vi "Set_Speed.vi"(5 "Channel Name (Calib Tweak)":string, 6 "Calib Tweak":dbl format="%.2f", 7 "Client Name":string, 8 "Channel Name (Volts/Amps)":string, 9 "Demanded Velocity":dbl format="%.2f", 10 "Channel Name (Velocity)":string) -> ()   [LabVIEW 2012]
uses:
  ADAM Client/Sub VIs/ADAM Controls/Update_scan_value.ctl
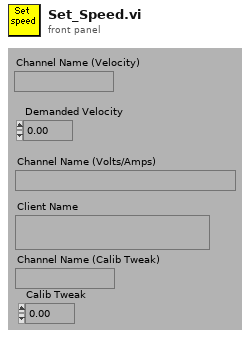
[diagram p1: front panel]
types:
  T1 = enum16{"Append to Global", "Read Global then Clear"}
  T2 = typedef "Update_scan_value.ctl" = cluster{"Channel Name":string, "New Value":dbl}
  T3 = typedef "Ch_description_ADAM.ctl" = cluster{"Ch Name":string, "Type":T4, "Function":T5, "Ch State":T6, "Calibration type":T7, "A":dbl, "B":dbl, "C":dbl, "D":dbl, "Comments":string, "Address":T8, "String":string, "Duty":u16}
  T4 = typedef "Module_type_ADAM.ctl" = string
  T5 = typedef "Function_ADAM.ctl" = enum16{"Analogue Input", "Digital Input", "Event counter", "Event rate", "Analogue Output", "Digital Output", "Relay Output"}
  T6 = typedef "Channel_State.ctl" = enum16{"On", "Off", "Always On", "Always Off"}
  T7 = typedef "Calib_type_ADAM.ctl" = enum16{"Raw", "Bx + A", "Cx^2 + Bx + A", "Dx^3 + Cx^2 + Bx + A", "In Band", "Hi-Tec Q", "Hi-Tec M_dot", "Text"}
  T8 = typedef "Address.ctl" = cluster{"Main":i32, "Ch.":i32, "Sub":i32, "Port Name":string}
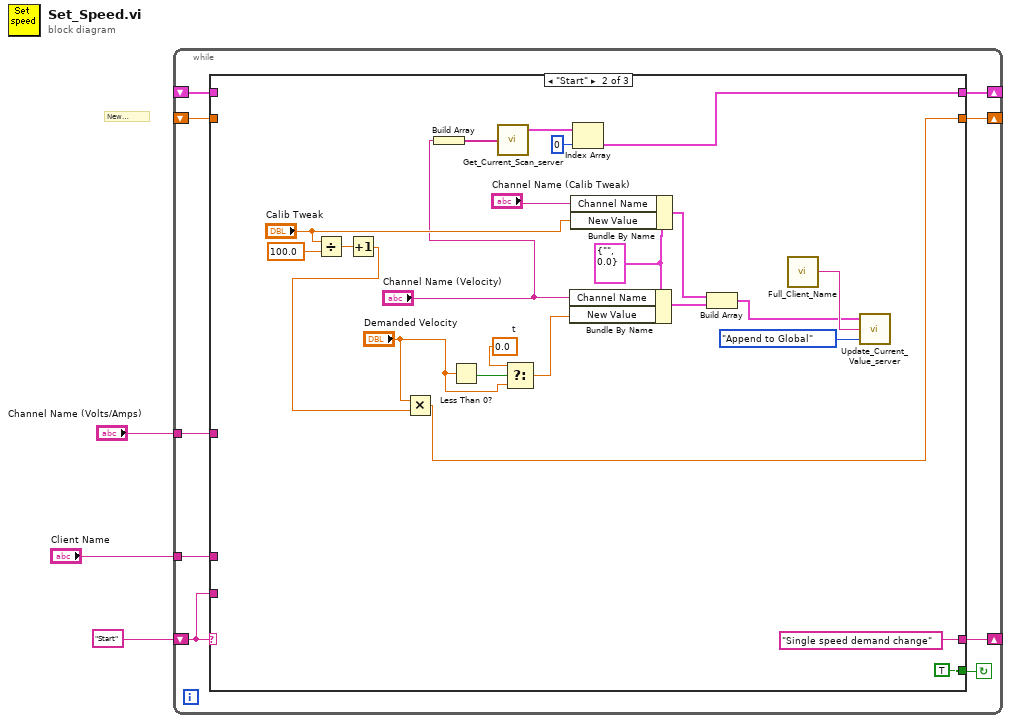
[diagram p0: block diagram]
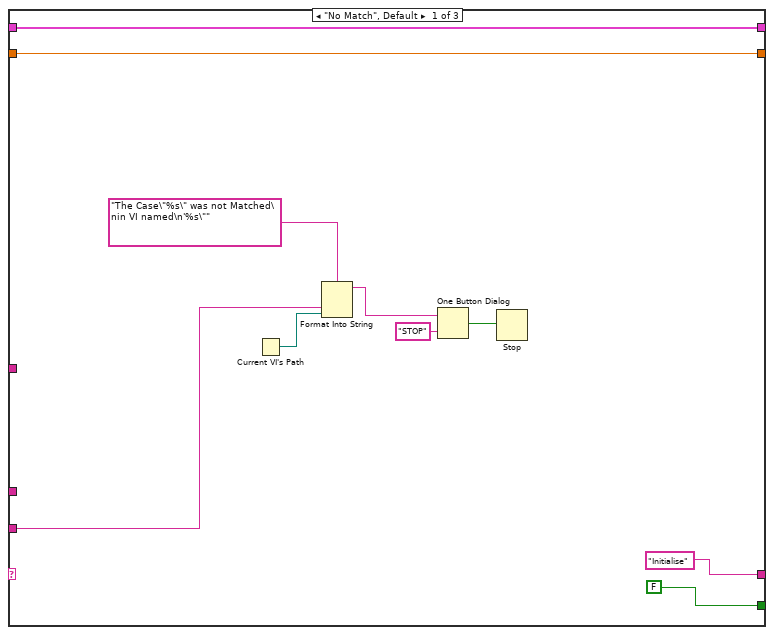
[diagram p2: hidden frame]
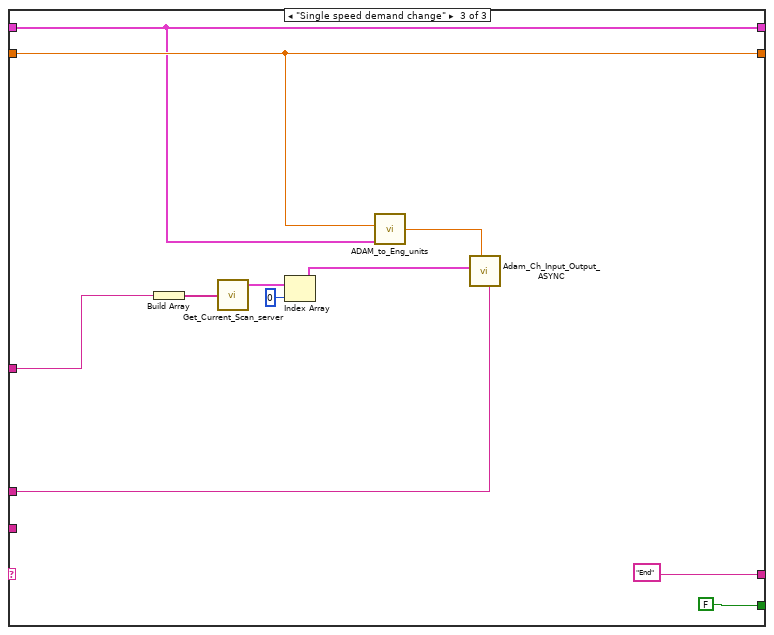
[diagram p3: hidden frame]
diagram:
  # "New Demand"
  n1 = while {
    shift-left: "Start" -> [w10]
    shift-right: [w11] -> _
    shift-right: [w7] -> _
    shift-left: _ -> [w8]
    tunnel: "Channel Name (Volts/Amps)" -> [w9]
    tunnel: "Client Name" -> [w6]
    shift-right: [w5] -> _
    shift-left: _ -> [w4]
    stop <- w12 continue-if-true
    n2 = case shown="\"Start\"" w10 {
      tunnel: [FALSE TRUE FALSE] -> w12
      tunnel: ["Initialise" "Single speed demand change" "End"] -> w11
      tunnel: w10 -> [w17 _ _]
      tunnel: w9 -> [_ _ w51]
      tunnel: w8 -> [w14 _ w48]
      tunnel: [w14 w30 w48] -> w7
      tunnel: w6 -> [_ _ w50]
      tunnel: [w13 w25 w46] -> w5
      tunnel: w4 -> [w13 _ w46]
      frame "No Match", Default {
        n3 = Current VI's Path() -> (path=w16:path)
        n4 = Format Into String(format string="The Case\"%s\" was not Matched\nin VI named\n'%s\"" ("Format String"), w17, w16) -> (resulting string=w20:string)  [unwired: 2 in, 1 out]
        n5 = One Button Dialog(message=w20, button name ("OK")="STOP") -> (true=w18:bool)
        n6 = Stop(stop? (T)=w18) -> ()
      }
      frame "Start" {
        w36 = T2 {"Channel Name"="", "New Value"=0.0} ("Update Scan Value Cluster")
        w42 = 0.0  # t
        n7 = Divide(x="Calib Tweak", y=100.0) -> (x/y=w41:dbl)
        n8 = Increment(x=w41) -> (x+1=w44:dbl)
        n9 = Multiply(x="Demanded Velocity", y=w44) -> (x*y=w30:dbl)
        n10 = Build Array("Channel Name (Velocity)") -> (w29:string[])
        n11 = Less Than 0?(x="Demanded Velocity") -> (x < 0?=w34:bool)
        n12 = call "Get_Current_Scan_server.vi"("Desired Channels"=w29) -> ("Ch Description Array"=w26:T3[])  [unwired: 2 out]
        n13 = Select(t=w42, s=w34, f="Demanded Velocity") -> (s? t:f=w43:dbl)
        n14 = Bundle By Name(cluster=w36, "Channel Name"="Channel Name (Velocity)", "New Value"=w43) -> (w32:T2)
        n15 = Bundle By Name(cluster=w36, "Channel Name"="Channel Name (Calib Tweak)", "New Value"="Calib Tweak") -> (w38:T2)
        n16 = Index Array(array=w26, index=0) -> (element=w25:T3)
        n17 = Build Array(w38, w32) -> (w33:T2[])
        n18 = call "Full_Client_Name.vi"() -> ("Client Name"=w35:string)
        n19 = call "Update_Current_Value_server.vi"("Mode"=T1."Append to Global", "Client HD name"=w35, "Update array in"=w33) -> ()  [unwired: 1 out]
      }
      frame "Single speed demand change" {
        n20 = Build Array(w51) -> (w54:string[])
        n21 = call "Get_Current_Scan_server.vi"("Desired Channels"=w54) -> ("Ch Description Array"=w52:T3[])  [unwired: 2 out]
        n22 = Index Array(array=w52, index=0 ("Index")) -> (element=w49:T3)
        n23 = call "ADAM_to_Eng_units.vi"("Ch Description"=w46, "Raw"=w48) -> ("Calibrated units"=w47:dbl)  [unwired: 4 out]
        n24 = call "Adam_Ch_Input_Output_ASYNC.vi"("Client Name"=w50, "Value to Output"=w47, "Ch Discription"=w49) -> ()  [unwired: 4 in, 5 out]
      }
    }
  }
